vi "(SubVI) Temp dependent of Viscosity of water_YCC.vi"(4 "Temperature (C)":dbl) -> (1 "Viscosity (mPa*s)":dbl)   [LabVIEW 2014]
uses:
  <vilib>/Analysis/polynomials.llb/Scalar Polynomial Evaluation (DBL).vi
  <vilib>/Analysis/NI_AALPro.lvlib
panel:
  out "XY Graph":cluster{"X":dbl[], "Y":dbl[]}[](graph)
  out "Viscosity (mPa*s)":dbl[](array[numeric])
  out "Temperature (C)":dbl[](array[numeric])
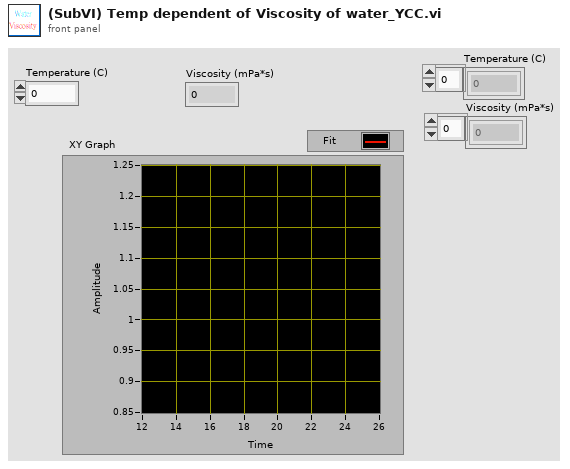
[diagram p1: front panel]
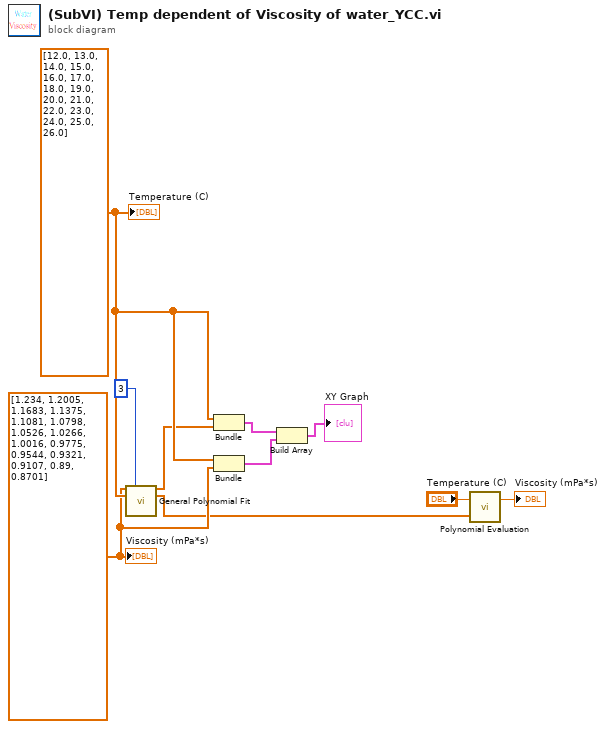
[diagram p0: block diagram]
diagram:
  w9 = dbl[] [1.234, 1.2005, 1.1683, 1.1375, 1.1081, 1.0798, 1.0526, 1.0266, 1.0016, 0.9775, 0.9544, 0.9321, 0.9107, 0.89, 0.8701] ("Y")
  w10 = dbl[] [12.0, 13.0, 14.0, 15.0, 16.0, 17.0, 18.0, 19.0, 20.0, 21.0, 22.0, 23.0, 24.0, 25.0, 26.0] ("X")
  n1 = call <vilib>:"General Polynomial Fit.vi"("Y"=w9, "polynomial order"=3, "X"=w10) -> ("Best Polynomial Fit"=w8:dbl[], "Polynomial Coefficients"=w3:dbl[])  [unwired: 9 in, 2 out]
  n2 = Bundle("X"=w10, "Best Polynomial Fit"=w8) -> (w7:cluster{"X":dbl[], "Best Polynomial Fit":dbl[]})  [unwired: 1 in]
  n3 = Bundle("X"=w10, "Y"=w9) -> (w6:cluster{"X":dbl[], "Y":dbl[]})  [unwired: 1 in]
  n4 = Build Array(w7, w6) -> (→"XY Graph":cluster{"X":dbl[], "Y":dbl[]}[])
  n5 = call-poly <vilib>:"Polynomial Evaluation.vi"("P(x)"=w3, "a"="Temperature (C)") -> ("P(a)"=→"Viscosity (mPa*s)":dbl)  [unwired: 1 out]
  "Temperature (C)" <- w10
  "Viscosity (mPa*s)" <- w9
